vi "odczyt pliku z temp.vi"(0 "error in (no error)":errorcluster) -> (1 "Nagłówki (tablica 1D)":string[](array[string]), 2 "Temperatury (wybrany kanał)":dbl[](array[numeric]), 3 "Kolumna z czasem (tablica 1D)":string[](array[string]), 4 "error out":errorcluster)   [LabVIEW 2009]
uses:
  <vilib>/Utility/file.llb/Read From Spreadsheet File (string).vi
panel:
  in  "Akceptuj":bool
  in  "Temperatura na zdjęcia z:":u16(ring) items=["Stolik", "Kroplówka", "Obok", "Termopara_K"]
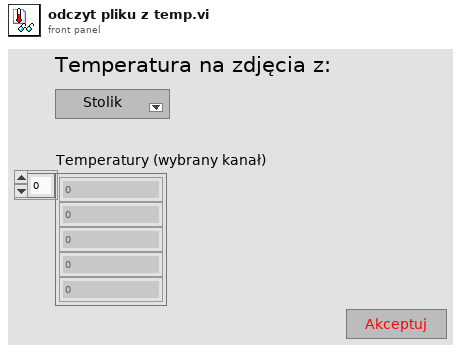
[diagram p1: front panel]
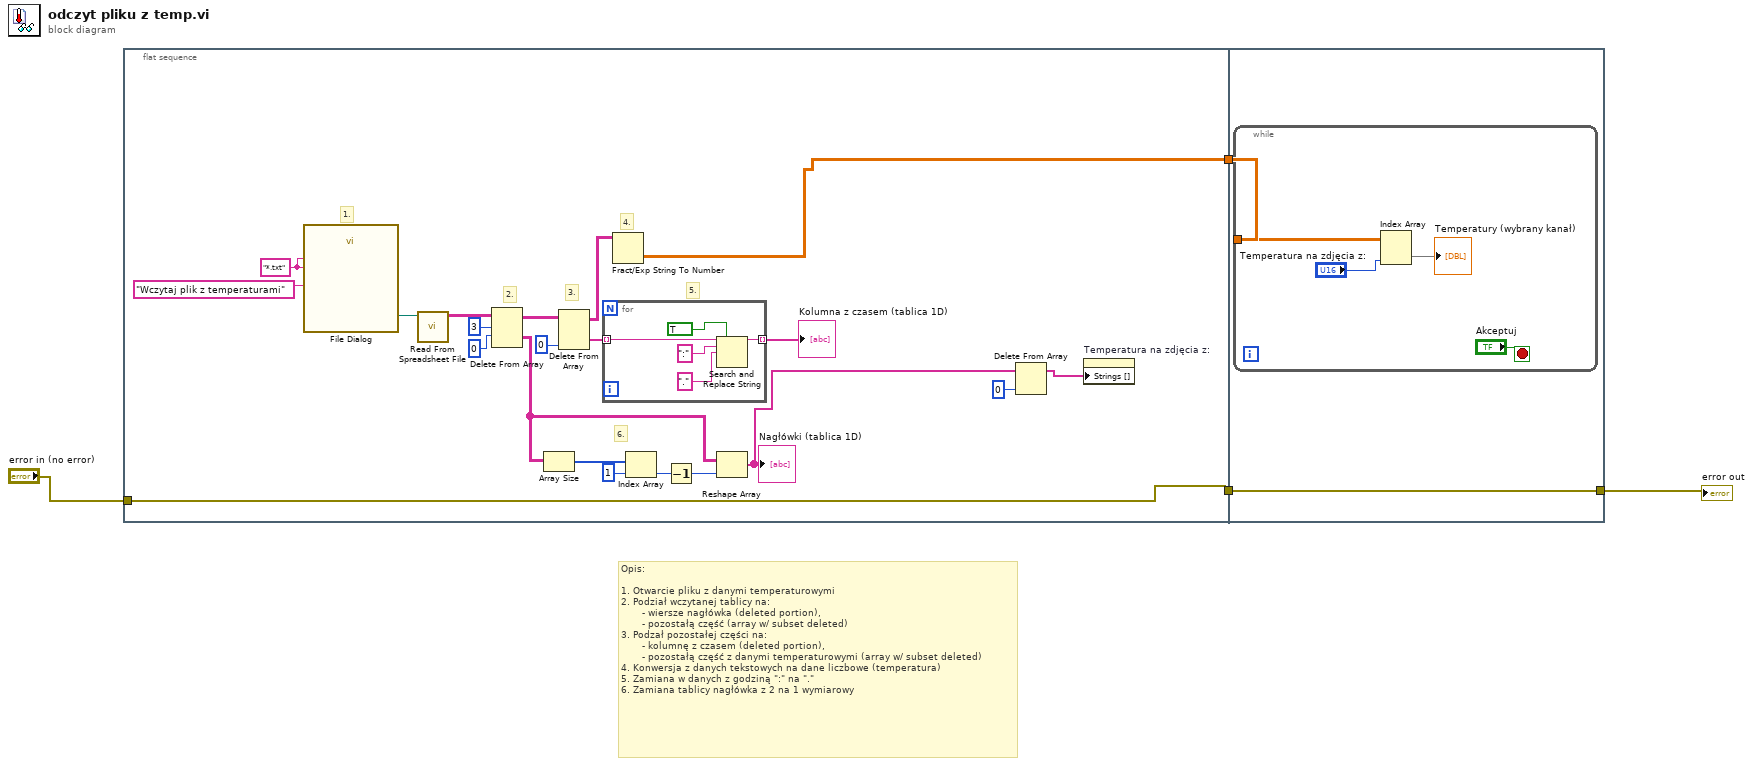
[diagram p0: block diagram]
diagram:
  # "Opis:\n\n1. Otwarcie pliku z danymi temperaturowymi\n2. Podział wczytanej tablicy na:\n       - wiersze nagłówka (deleted portion),\n       - pozostałą część (array w/ subset deleted) \n3. Podzał pozostałej części na:\n       - kolumnę z czasem (deleted portion),\n       - pozostałą część z danymi temperaturowymi (array w/ subset deleted) \n4. Konwersja z danych tekstowych na dane liczbowe (temperatura)\n5. Zamiana w danych z godziną \":\" na \".\"\n6. Zamiana tablicy nagłówka z 2 na 1 wymiarowy"
  n1 = flat-sequence {
    tunnel: [w9] -> w4
    tunnel: [w5] -> w3
    tunnel: "error in (no error)" -> [w5]
    tunnel: w4 -> [w32]
    tunnel: w3 -> [w31]
    tunnel: [w31] -> w1
    frame #0 {
      w23 = "*.txt" ("pattern label")
      # "6."
      # "5."
      # "4."
      # "3."
      # "2."
      # "1."
      n2 = call "File Dialog"("prompt"="Wczytaj plik z temperaturami", "pattern (all files)"=w23, "pattern label"=w23) -> ("selected path"=w25:path)  [unwired: 9 in, 3 out]
      n3 = call-poly <vilib>:"Read From Spreadsheet File.vi"("file path (dialog if empty)"=w25) -> ("all rows"=w22:string[][])  [unwired: 6 in, 4 out]
      n4 = Delete From Array(array=w22, length=3, index (row)=0) -> (deleted portion=w16:string[][], array with subset deleted=w19:string[][])  [unwired: 1 in]
      n5 = Array Size(array=w16) -> (size(s)=w15:i32[])
      n6 = Delete From Array(array=w19, index (col)=0 ("disabled index (col)")) -> (deleted portion=w11:string[], array with subset deleted=w17:string[][])  [unwired: 2 in]
      n7 = for {
        tunnel: w11 -> [w30] mode=indexing
        tunnel: [w29] -> w10 mode=indexing
        n8 = Search and Replace String(replace all?=TRUE ("replace all? (F)"), input string=w30, search string=":", replace string="." ("replace string (\"\")")) -> (result string=w29:string)  [unwired: 4 in, 3 out]
      }
      "Kolumna z czasem (tablica 1D)" <- w10
      n9 = Fract/Exp String To Number(string=w17) -> (number=w9:dbl[][])  [unwired: 3 in, 1 out]
      n10 = Index Array(array=w15, index=1) -> (element=w14:i32)
      n11 = Decrement(x=w14) -> (x-1=w12:i32)
      n12 = Reshape Array(w16, w12) -> (w7:string[])
      "Nagłówki (tablica 1D)" <- w7
      n13 = Delete From Array(array=w7, index=0) -> (array with subset deleted=w6:string[])  [unwired: 1 in, 1 out]
      n14 = property on="Temperatura na zdjęcia z:" class="Ring (strict)"("Strings []"=w6) -> ()  [unwired: 2 in, 2 out]
    }
    frame #1 {
      n15 = while {
        tunnel: w32 -> [w34]
        stop <- "Akceptuj" stop-if-true
        n16 = Index Array(array=w34, index (col)="Temperatura na zdjęcia z:") -> (element=→"Temperatury (wybrany kanał)":dbl[])  [unwired: 1 in]
      }
    }
  }
  "error out" <- w1
